vi "Initiate multi-module assembly.vi"(0 "Database Entry in":refnum<class "Database Entry.lvclass">, 11 "error in (no error)":errorcluster) -> (2 "Feet check":bool, 4 "Database Entry out":refnum<class "Database Entry.lvclass">, 6 "Module?":bool, 8 "Abort out":bool, 14 "Module type out":string, 15 "error out":errorcluster)   [LabVIEW 2021, in "Database Entry.lvclass"]
uses:
  Database Entry.lvclass
  Database Entry.lvclass/Database Entry.ctl
  Components/Stack/Stack.lvclass
  <vilib>/Utility/file.llb/Read Delimited Spreadsheet (string).vi
  SubVIs/assembly_tray_region.vi
panel:
  in  "De/Select All":bool
  in  "Set default module type":bool
  out "Now assembling...":string
  in  "Abort":bool
  in  "Relative humidity":dbl
  in  "Temperature (C)":dbl
  in  "Adhesive":u16(ring) items=["Hybrid", "Transfer tape only", "Epoxy only"]
  in  "Module Type":u16(ring) items=["CMU,LD,Full,200,CuW", "CMU,LD,Full,300,CuW", "CMU,LD,Full,300,Ti", "CMU,LD,Full,200,CF", "CMU,LD,Full,300,CF"]
  in  "Operator":u16(ring) items=["jestein", "japicard", "simurthy", "atawker", "cmumac"]
  in  "Select positions for assembly":cluster{"1":bool, "2":bool, "3":bool, "4":bool}
  in  "Submit":bool
  # "Tray Slot 1"
  # "Tray Slot 2"
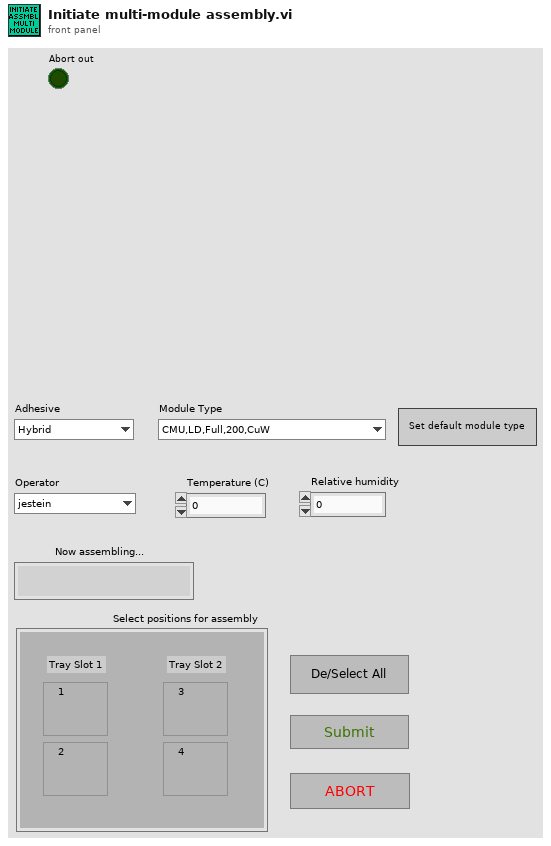
[diagram p1: front panel]
types:
  T1 = typedef "File Paths.ctl" = cluster{"Glue Pattern Folder":path, "Carrier Tray Folder":path, "Pick Up Tool Fixture Folder":path, "Components Folder":path, "Bellows Tool Offset.txt":path, "Pick Up Tool Offset.txt":path, "Dispense Tip Offset.txt":path, "Log Files":path, "Gantry Assembly Map.txt":path, "Syringe and offset map.txt":path, "Controllers Folder":path, "Local dbase config":path}
  T2 = cluster{"[0]":bool, "[1]":bool, "[2]":bool, "[3]":bool}
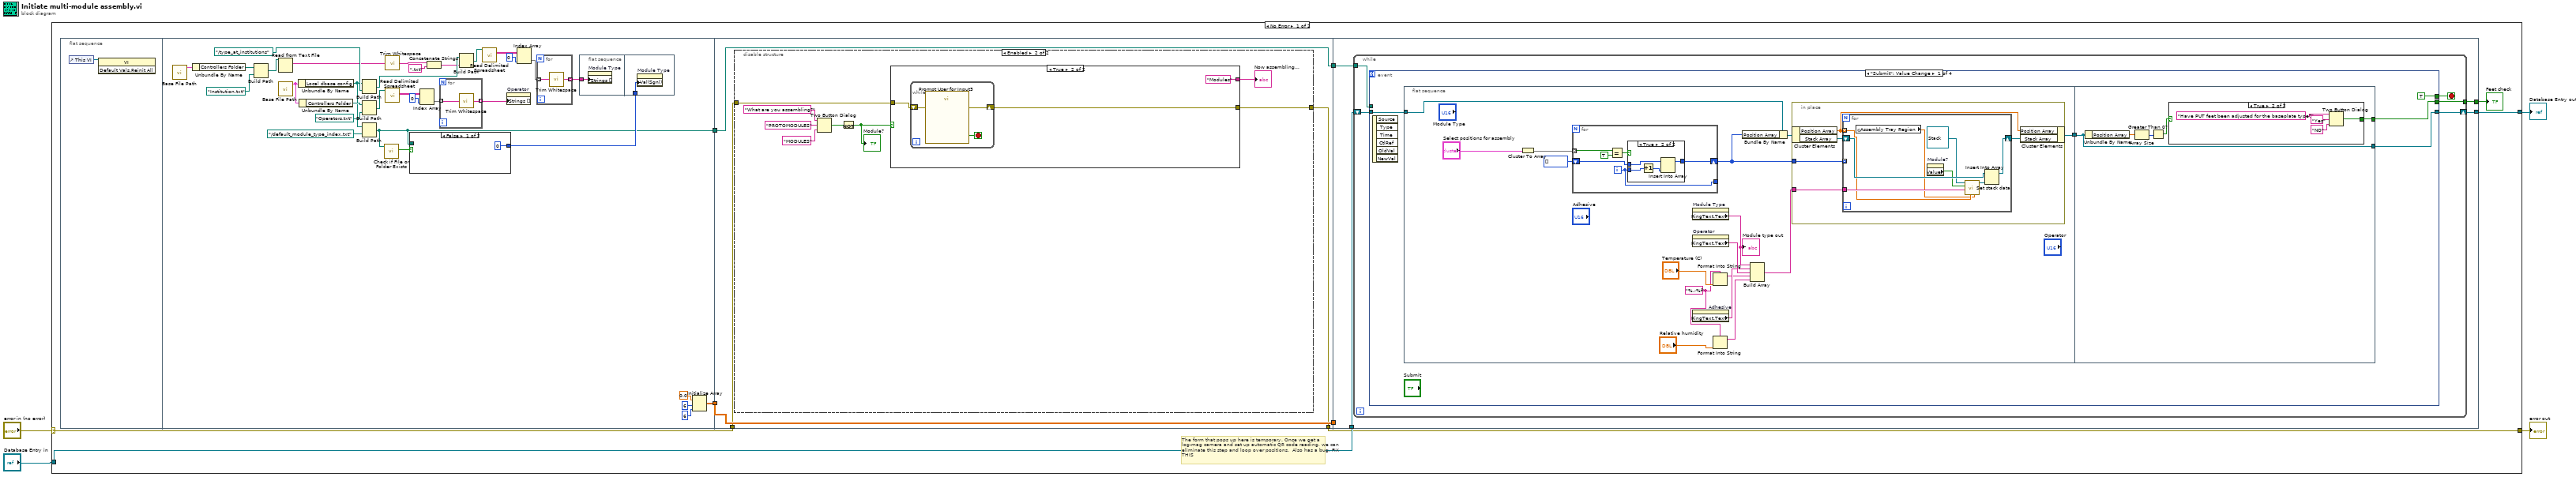
[diagram p0: block diagram]
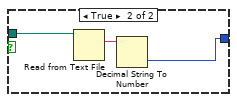
[diagram p2: hidden frame]
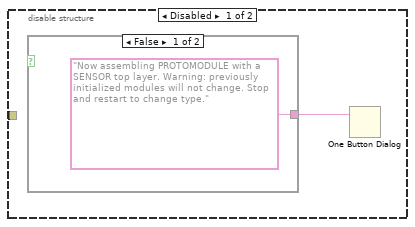
[diagram p3: hidden frame]
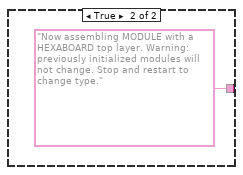
[diagram p4: hidden frame]
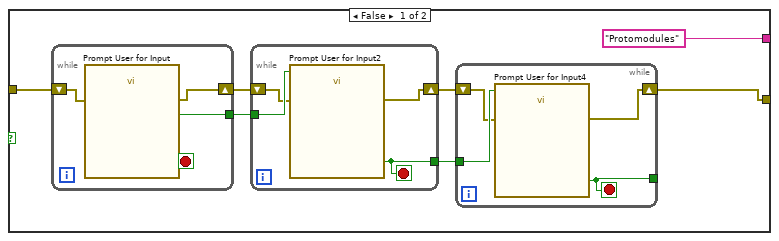
[diagram p5: hidden frame]
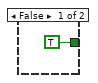
[diagram p7: hidden frame]
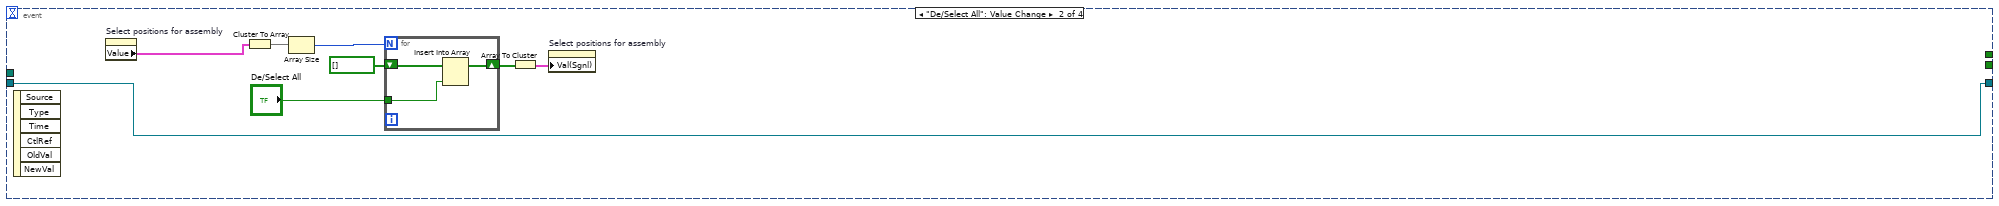
[diagram p8: hidden frame]
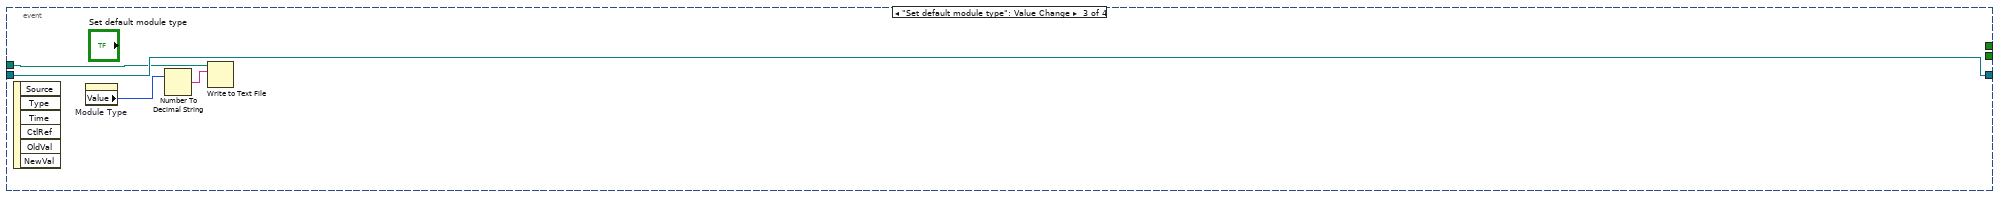
[diagram p9: hidden frame]
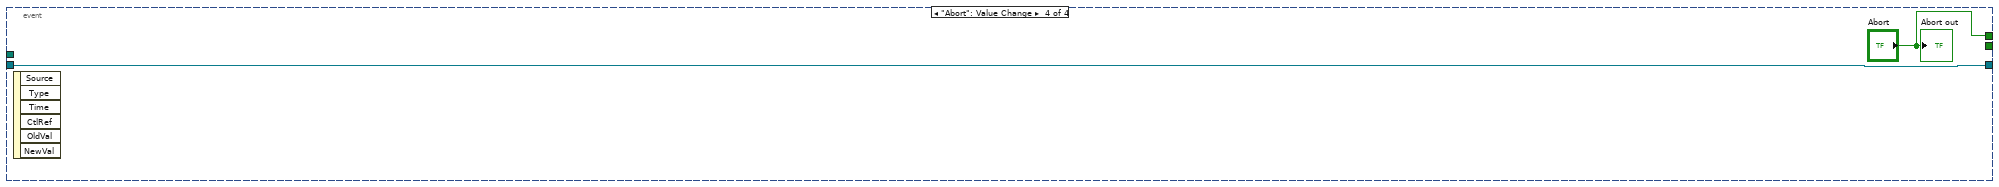
[diagram p10: hidden frame]
diagram:
  n1 = case shown="No Error" "error in (no error)" {
    selector: "error in (no error)" -> [w6 w178]
    tunnel: [w5 w178] -> w3
    tunnel: [w9 w177] -> w1
    tunnel: "Database Entry in" -> [w13 w177]
    frame No Error {
      # "The form that pops up here is temporary. Once we get a log-mag camera and set up automatic QR code reading, we can eliminate this step and loop over positions.  Also has a bug. FIX THIS"
      n2 = flat-sequence {
        tunnel: [w39] -> w11
        tunnel: [w15] -> w8
        tunnel: w11 -> [w60]
        tunnel: [w60] -> w10
        tunnel: w8 -> [w59]
        tunnel: [w59] -> w7
        tunnel: w6 -> [w58]
        tunnel: [w57] -> w5
        tunnel: w10 -> [_]
        tunnel: w13 -> [w99]
        tunnel: [w98] -> w9
        tunnel: [w97] -> w12
        tunnel: w7 -> [w96]
        frame #0 {
          n3 = control-ref of="This VI"() -> (w14:refnum<vi>)
          n4 = invoke class="VI" method="Default Vals.Reinit All"(reference=w14) -> ()  [unwired: 2 in, 3 out]
        }
        frame #1 {
          n5 = call "Base File Path.vi"() -> ("Paths Out"=w46:T1)  [unwired: 11 in]
          n6 = Unbundle By Name(w46) -> ("Controllers Folder"=w31:path)
          n7 = Build Path(base path=w31, name or relative path=path "Institution.txt") -> (appended path=w22:path)
          n8 = Read from Text File(file (use dialog)=w22) -> (text=w24:string)  [unwired: 3 in, 3 out]
          n9 = call "Base File Path.vi"() -> ("Paths Out"=w35:T1)  [unwired: 11 in]
          n10 = Unbundle By Name(w35) -> ("Local dbase config"=w17:path)
          n11 = Unbundle By Name(w35) -> ("Controllers Folder"=w44:path)
          n12 = Build Path(base path=w17, name or relative path=path "../type_at_institutions") -> (appended path=w32:path)
          n13 = Build Path(base path=w44, name or relative path=path "Operators.txt") -> (appended path=w42:path)
          n14 = Build Path(base path=w17, name or relative path=path "../default_module_type_index.txt") -> (appended path=w15:path)
          n15 = call <vilib>:"Check if File or Folder Exists.vi"("path"=w15) -> ("file or folder exists?"=w18:bool)  [unwired: 8 in, 2 out]
          n16 = call <vilib>:"Trim Whitespace.vi"("string"=w24) -> ("trimmed string"=w21:string)  [unwired: 1 in]
          n17 = call-poly <vilib>:"Read Delimited Spreadsheet.vi"("file path (dialog if empty)"=w42) -> ("all rows"=w41:string[][])  [unwired: 9 in, 5 out]
          n18 = case shown="False" w18 {
            tunnel: w15 -> [_ w50]
            tunnel: [0 w48] -> w23
            frame False {
            }
            frame True {
              n19 = Read from Text File(file (use dialog)=w50) -> (text=w49:string)  [unwired: 3 in, 3 out]
              n20 = Decimal String To Number(string=w49) -> (number=w48:i32)  [unwired: 2 in, 1 out]
            }
          }
          n21 = Index Array(array=w41, index (col)=0 ("disabled index (col)")) -> (element=w27:string[])  [unwired: 1 in]
          n22 = Concatenate Strings(w21, ".txt" ("string")) -> (w29:string)
          n23 = for {
            tunnel: w27 -> [w56] mode=indexing
            tunnel: [w55] -> w26 mode=indexing
            n24 = call <vilib>:"Trim Whitespace.vi"("string"=w56) -> ("trimmed string"=w55:string)  [unwired: 1 in]
          }
          n25 = Build Path(base path=w32, name or relative path=w29) -> (appended path=w20:path)
          n26 = call-poly <vilib>:"Read Delimited Spreadsheet.vi"("file path (dialog if empty)"=w20) -> ("all rows"=w28:string[][])  [unwired: 9 in, 5 out]
          n27 = property on="Operator" class="Ring (strict)"("Strings []"=w26) -> ()  [unwired: 2 in, 2 out]
          n28 = Index Array(array=w28, index (col)=0 ("disabled index (col)")) -> (element=w19:string[])  [unwired: 1 in]
          n29 = for {
            tunnel: w19 -> [w54] mode=indexing
            tunnel: [w53] -> w25 mode=indexing
            n30 = call <vilib>:"Trim Whitespace.vi"("string"=w54) -> ("trimmed string"=w53:string)  [unwired: 1 in]
          }
          n31 = flat-sequence {
            tunnel: w25 -> [w51]
            tunnel: w23 -> [w52]
            frame #0 {
              n32 = property on="Module Type" class="Ring (strict)"("Strings []"=w51) -> ()  [unwired: 2 in, 2 out]
            }
            frame #1 {
              n33 = property on="Module Type" class="Ring (strict)"("Val(Sgnl)"=w52) -> ()  [unwired: 2 in, 2 out]
            }
          }
          n34 = Initialize Array(0.0 ("element"), 6 ("dimension size"), 6 ("dimension size")) -> (w39:dbl[][])
        }
        frame #2 {
          n35 = disable-structure shown="Enabled" {
            disable-tunnel: w58 -> [_ w65]
            disable-tunnel: [_ w64] -> w57
            frame Disabled {
              n36 = case shown="False" {
                selector: _ -> [_ _]
                tunnel: ["Now assembling PROTOMODULE with a SENSOR top layer. Warning: previously initialized modules will not change. Stop and restart to change type." "Now assembling MODULE with a HEXABOARD top layer. Warning: previously initialized modules will not change. Stop and restart to change type."] -> w61
                frame False {
                }
                frame True {
                }
              }
              n37 = One Button Dialog(message=w61) -> ()  [unwired: 1 in, 1 out]
            }
            frame Enabled {
              n38 = Two Button Dialog(message="What are you assembling?", 1:"MODULES" ("F button name (\"Cancel\")"), 2:"PROTOMODULES" ("T button name (\"OK\")")) -> (T button?=w68:bool)
              n39 = Not(x=w68) -> (.not. x?=w67:bool)
              "Module?" <- w67
              n40 = case shown="True" w67 {
                tunnel: ["Protomodules" ("Now assembling...") "Modules" ("Now assembling...")] -> w66
                tunnel: w65 -> [w73 w90]
                tunnel: [w72 w91] -> w64
                frame False {
                  n41 = while {
                    tunnel: [w89] -> w77
                    shift-right: [w88] -> w75
                    shift-left: w73 -> [w87]
                    stop <- w89 stop-if-true
                    n42 = call "Prompt User for Input"("error in (no error)"=w87) -> ("BPs ready?"=w89:bool, "error out"=w88:errorcluster)  [unwired: 16 in, 1 out]
                  }
                  n43 = while {
                    tunnel: w77 -> [w86]
                    tunnel: [w85] -> w76
                    shift-right: [w83] -> w74
                    shift-left: w75 -> [w84]
                    stop <- w85 stop-if-true
                    n44 = call "Prompt User for Input2"("Enable"=w86, "error in (no error)"=w84) -> ("Sensor tooling ready?"=w85:bool, "error out"=w83:errorcluster)  [unwired: 15 in, 1 out]
                  }
                  n45 = while {
                    tunnel: [w82] -> _
                    tunnel: w76 -> [w81]
                    shift-right: [w79] -> w72
                    shift-left: w74 -> [w80]
                    stop <- w82 stop-if-true
                    n46 = call "Prompt User for Input4"("Enable"=w81, "error in (no error)"=w80) -> ("No gaps?"=w82:bool, "error out"=w79:errorcluster)  [unwired: 15 in, 1 out]
                  }
                }
                frame True {
                  n47 = while {
                    shift-right: [w94] -> w91
                    shift-left: w90 -> [w93]
                    stop <- w95 stop-if-true
                    n48 = call "Prompt User for Input3"("error in (no error)"=w93) -> ("HB tooling ready?"=w95:bool, "error out"=w94:errorcluster)  [unwired: 16 in, 1 out]
                  }
                }
              }
              "Now assembling..." <- w66
            }
          }
        }
        frame #3 {
          n49 = while {
            shift-right: [w104] -> w98
            shift-left: w99 -> [w103]
            tunnel: [w101] -> w97
            tunnel: w96 -> [w100]
            stop <- w102 stop-if-true
            n50 = event shown="[0] \"Submit\": Value Change" {
              selector: _ -> [_ _ _ _]
              dyn-events: _ -> [_ _ _ _]
              timeout: _ -> [_ _ _ _]
              tunnel: [TRUE ("T button?") _ _ "Abort"] -> w102
              tunnel: w103 -> [w107 w160 w174 w175]
              tunnel: [w105 w160 w174 w175] -> w104
              tunnel: [w108 _ _ _] -> w101
              tunnel: w100 -> [_ _ w171 _]
              event "Submit": Value Change {
                n51 = event-data() -> ()  [unwired: 1 in, 6 out]
                n52 = flat-sequence {
                  tunnel: w107 -> [w122]
                  tunnel: [w117] -> w106
                  tunnel: [w154] -> w108
                  tunnel: w106 -> [w150]
                  tunnel: [w150] -> w105
                  frame #0 {
                    w110 = "%.;%f" ("format string")
                    n53 = Cluster To Array(cluster="Select positions for assembly") -> (array=w125:bool[])
                    n54 = for {
                      shift-right: [w141] -> w119
                      shift-left: i32[] [] -> [w142]
                      tunnel: [w140] -> _
                      tunnel: w125 -> [w139] mode=indexing
                      i -> [w140]
                      n55 = Equal?(x=w139, y=TRUE) -> (x = y?=w143:bool)
                      n56 = case shown="True" w143 {
                        tunnel: w142 -> [w145 w148]
                        tunnel: w140 -> [_ w147]
                        tunnel: [w145 w146] -> w141
                        frame False {
                        }
                        frame True {
                          n57 = Increment(x=w147) -> (x+1=w149:i32)
                          n58 = Insert Into Array(array=w148, new element=w149) -> (w146:i32[])  [unwired: 1 in]
                        }
                      }
                    }
                    n59 = property on="Module Type" class="Ring (strict)"() -> ("RingText.Text"=w115:string)  [unwired: 2 in, 2 out]
                    "Module type out" <- w115
                    n60 = property on="Operator" class="Ring (strict)"() -> ("RingText.Text"=w121:string)  [unwired: 2 in, 2 out]
                    n61 = property on="Adhesive" class="Ring (strict)"() -> ("RingText.Text"=w120:string)  [unwired: 2 in, 2 out]
                    n62 = Format Into String(format string=w110, "Temperature (C)") -> (resulting string=w113:string)  [unwired: 2 in, 1 out]
                    n63 = Format Into String(format string=w110, "Relative humidity") -> (resulting string=w111:string)  [unwired: 2 in, 1 out]
                    n64 = Bundle By Name(cluster=w122, "Position Array"=w119) -> (w118:refnum<class "Database Entry.lvclass">)
                    n65 = Build Array(w115, w120, w121, w113, w111) -> (w116:string[])
                    n66 = in-place {
                      in-place-border: w119 -> [w130]
                      in-place-border: w116 -> [w127]
                      n67 = in-place-cluster #1(w118) -> ("Position Array"=w126:dbl[], "Stack Array"=w129:refnum<class "Stack.lvclass">[])
                      n68 = for {
                        tunnel: w130 -> [_] mode=indexing
                        shift-right: [w137] -> w128
                        shift-left: w129 -> [w138]
                        tunnel: w127 -> [w134]
                        tunnel: w126 -> [w132] mode=indexing
                        n69 = global read "assembly_tray_region.vi" "Assembly Tray Region"() -> (w131:dbl)
                        n70 = property on="Module?" class="Bool (strict)"() -> ("Value"=w133:bool)  [unwired: 2 in, 2 out]
                        n71 = call "Set stack data.vi"("Region"=w131, "Position"=w132, "Common data array"=w134, "Is module?"=w133, "Stack in"=refnum<class "Stack.lvclass"> refnum ("Stack.lvclass")) -> ("Stack out"=w135:refnum<class "Stack.lvclass">)  [unwired: 5 in, 1 out]
                        n72 = Insert Into Array(array=w138, new element=w135) -> (w137:refnum<class "Stack.lvclass">[])  [unwired: 1 in]
                      }
                      n73 = in-place-cluster #1("Position Array"=w126, "Stack Array"=w128) -> (w117:refnum<class "Database Entry.lvclass">)
                    }
                  }
                  frame #1 {
                    n74 = Unbundle By Name(w150) -> ("Position Array"=w153:dbl[])
                    n75 = Array Size(array=w153) -> (size(s)=w152:i32)
                    n76 = Greater Than 0?(x=w152) -> (x > 0?=w151:bool)
                    n77 = case shown="True" w151 {
                      tunnel: [TRUE ("T button?") w156] -> w154
                      frame False {
                      }
                      frame True {
                        n78 = Two Button Dialog(message="Have PUT feet been adjusted for the baseplate type?", 1:"NO" ("F button name (\"Cancel\")"), 2:"Yes" ("T button name (\"OK\")")) -> (T button?=w156:bool)
                      }
                    }
                  }
                }
              }
              event "De/Select All": Value Change {
                n79 = event-data() -> ()  [unwired: 1 in, 6 out]
                n80 = property on="Select positions for assembly" class="Clust (strict)"() -> ("Value"=w167:cluster{"1":bool, "2":bool, "3":bool, "4":bool})  [unwired: 2 in, 2 out]
                n81 = Cluster To Array(cluster=w167) -> (array=w166:bool[])
                n82 = Array Size(array=w166) -> (size(s)=w165:i32)
                n83 = for {
                  N: w165 -> [_]
                  shift-right: [w169] -> w163
                  shift-left: bool[] [] -> [w170]
                  tunnel: "De/Select All" -> [w168]
                  n84 = Insert Into Array(array=w170, new element=w168) -> (w169:bool[])  [unwired: 1 in]
                }
                n85 = Array To Cluster(array=w163) -> (cluster=w162:T2)
                n86 = property on="Select positions for assembly" class="Clust (strict)"("Val(Sgnl)"=w162) -> ()  [unwired: 2 in, 2 out]
              }
              event "Set default module type": Value Change {
                n87 = event-data() -> ()  [unwired: 1 in, 6 out]
                n88 = property on="Module Type" class="Ring (strict)"() -> ("Value"=w172:u16)  [unwired: 2 in, 2 out]
                n89 = Number To Decimal String(number=w172) -> (decimal integer string=w173:string)  [unwired: 1 in]
                n90 = Write to Text File(file (use dialog)=w171, text=w173) -> ()  [unwired: 2 in, 3 out]
              }
              event "Abort": Value Change {
                n91 = event-data() -> ()  [unwired: 1 in, 6 out]
                "Abort out" <- "Abort"
              }
            }
          }
        }
      }
      "Feet check" <- w12
    }
    frame Error {
    }
  }
  "error out" <- w3
  "Database Entry out" <- w1
